vi "Read Tracking Cluster.vi"(8 "error in (no error)":errorcluster, 11 "Supervisor in":refnum<class "Supervisor.lvclass">) -> (0 "error out":errorcluster, 2 "Tracking Cluster":T1, 3 "Supervisor out":refnum<class "Supervisor.lvclass">)   [LabVIEW 2014, in "Supervisor.lvclass"]
uses:
  Supervisor.lvclass
  Supervisor.lvclass/Supervisor.ctl
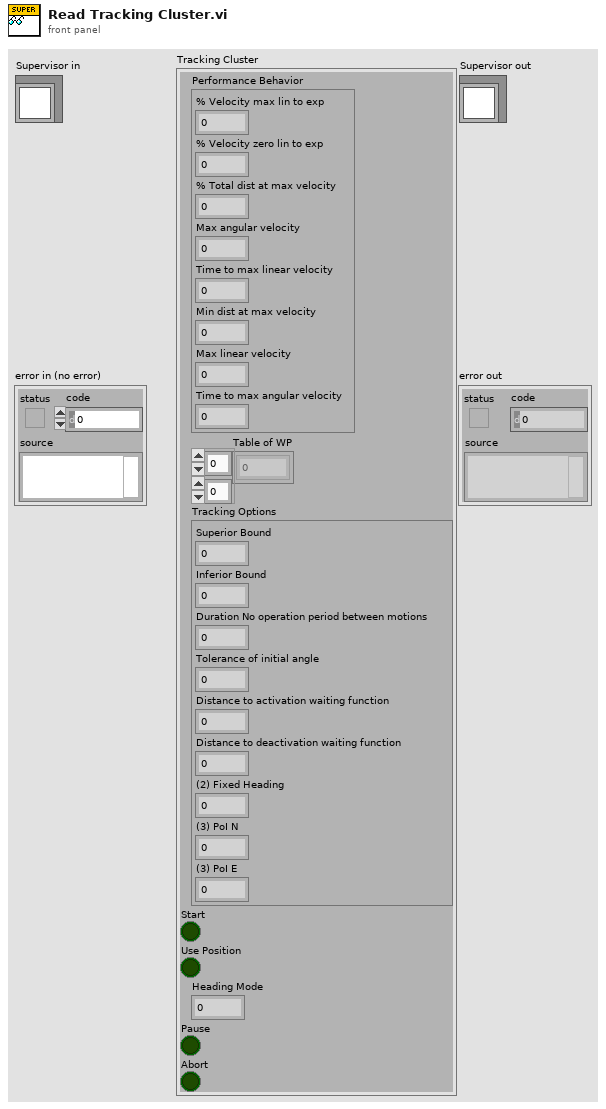
[diagram p1: front panel]
types:
  T1 = cluster{"Performance Behavior":cluster{"% Velocity max lin to exp":dbl, "% Velocity zero lin to exp":dbl, "% Total dist at max velocity":dbl, "Max angular velocity":dbl, "Time to max linear velocity":dbl, "Min dist at max velocity":dbl, "Max linear velocity":dbl, "Time to max angular velocity":dbl}, "Table of WP":dbl[][], "Tracking Options":cluster{"Superior Bound":dbl, "Inferior Bound":dbl, "Duration No operation period between motions":dbl, "Tolerance of initial angle":dbl, "Distance to activation waiting function":dbl, "Distance to deactivation waiting function":dbl, "(2) Fixed Heading":dbl, "(3) PoI N":dbl, "(3) PoI E":dbl}, "Start":bool, "Use Position":bool, "Heading Mode":u16, "Pause":bool, "Abort":bool}
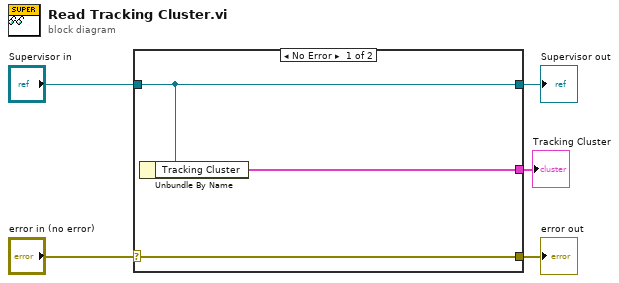
[diagram p0: block diagram]
diagram:
  n1 = case shown="No Error" "error in (no error)" {
    selector: "error in (no error)" -> [w8 w9]
    tunnel: [w8 w9] -> w4
    tunnel: [w7 w10] -> w2
    tunnel: "Supervisor in" -> [w7 w10]
    tunnel: [w6 _] -> w1
    frame No Error {
      n2 = Unbundle By Name(w7) -> ("Tracking Cluster"=w6:T1)
    }
    frame Error {
    }
  }
  "error out" <- w4
  "Supervisor out" <- w2
  "Tracking Cluster" <- w1
